vi "Create LVClass for Oneof.vi"(7 "Parent Message Typedef":refnum<vi>, 8 "error in (no error)":errorcluster, 9 "Message Elements":T1[](array[typedef]), 10 "Message Name":string, 11 "Library":refnum<vi>) -> (0 "error out":errorcluster, 3 "Library":refnum<vi>)   [LabVIEW 2019]
uses:
  TypeDefs/Message Element Metadata (Scripting).ctl
  TypeDefs/Message Element Type.ctl
  gRPC Template Creation Utility.lvlib
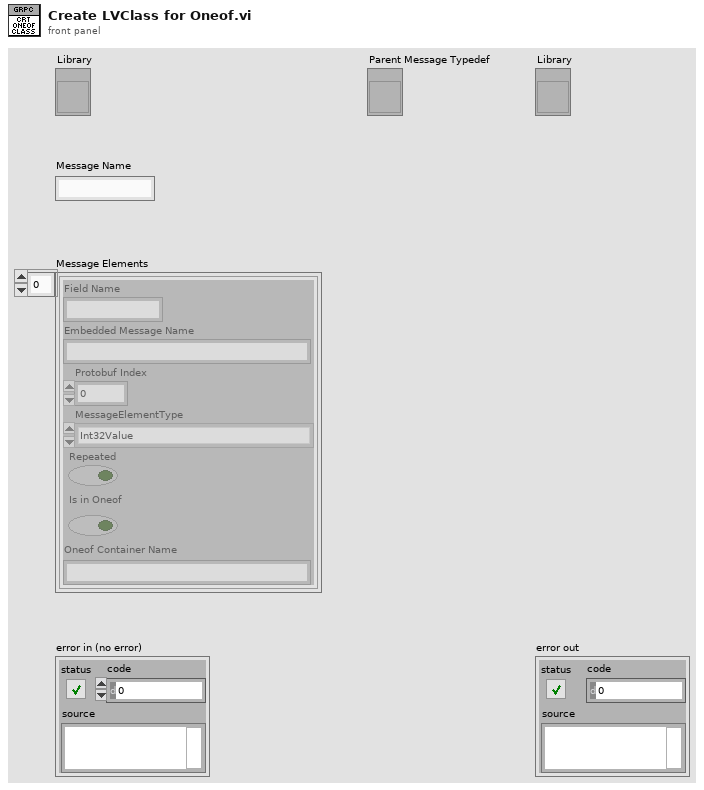
[diagram p1: front panel]
types:
  T1 = typedef "gRPC Template Creation Utility.lvlib/Message Element Metadata (Scripting).ctl" = cluster{"Field Name":string, "Embedded Message Name":string, "Protobuf Index":i32, "MessageElementType":T2, "Repeated":bool, "Is in Oneof":bool, "Oneof Container Name":string}
  T2 = typedef "gRPC Template Creation Utility.lvlib/Message Element Type.ctl" = enum32{"Int32Value", "FloatValue", "DoubleValue", "BoolValue", "StringValue", "MessageValue", "Int64Value", "UInt32Value", "UInt64Value", "EnumValue", "Bytes", "Fixed64", "Fixed32", "SFixed64", "SFixed32", "SInt64", "SInt32"}
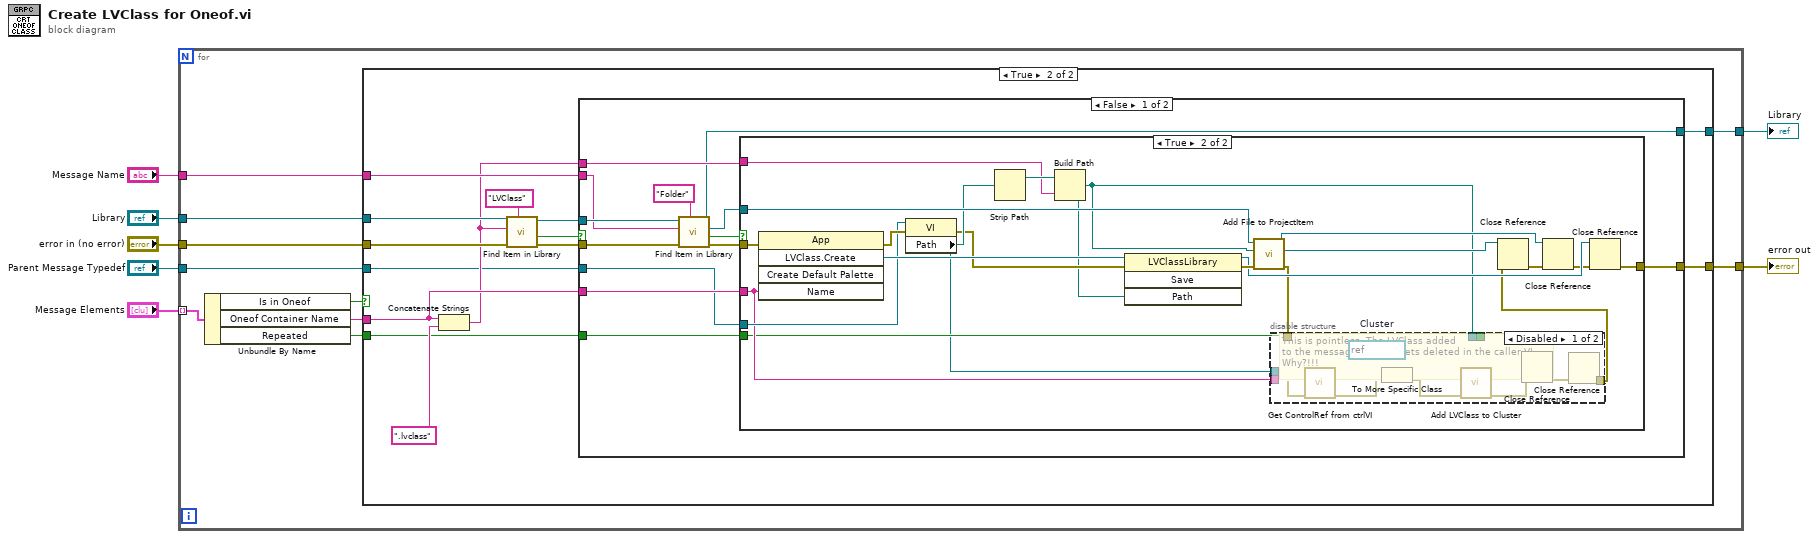
[diagram p0: block diagram]
diagram:
  n1 = for {
    tunnel: "Message Elements" -> [w17] mode=indexing
    tunnel: "error in (no error)" -> [w14]
    tunnel: [w13] -> w5
    tunnel: "Message Name" -> [w12]
    tunnel: "Library" -> [w11]
    tunnel: [w10] -> w2
    tunnel: "Parent Message Typedef" -> [w9]
    n2 = Unbundle By Name(w17) -> ("Is in Oneof"=w15:bool, "Oneof Container Name"=w16:string, "Repeated"=w8:bool)
    n3 = case shown="True" w15 {
      tunnel: [w19 w33] -> w13
      tunnel: w16 -> [_ w32]
      tunnel: w14 -> [w19 w29]
      tunnel: w12 -> [_ w31]
      tunnel: w11 -> [w18 w28]
      tunnel: [w18 w30] -> w10
      tunnel: w9 -> [_ w21]
      tunnel: w8 -> [_ w20]
      frame False {
      }
      frame True {
        n4 = Concatenate Strings(w32, ".lvclass" ("string")) -> (w25:string)
        n5 = call "Find Item in Library.vi"("Item Type"="LVClass", "error in (no error)"=w29, "Item Name"=w25, "Library item in"=w28) -> ("error out"=w23:errorcluster, "Found?"=w22:bool, "Library item out"=w27:refnum<vi>)  [unwired: 4 in, 1 out]
        n6 = case shown="False" w22 {
          tunnel: [w42 w86] -> w33
          tunnel: w32 -> [w41 _]
          tunnel: w31 -> [w36 _]
          tunnel: [w37 w87] -> w30
          tunnel: w27 -> [w38 w87]
          tunnel: w25 -> [w40 _]
          tunnel: w23 -> [w39 w86]
          tunnel: w21 -> [w35 _]
          tunnel: w20 -> [w34 _]
          frame False {
            n7 = call "Find Item in Library.vi"("Item Type"="Folder", "error in (no error)"=w39, "Item Name"=w36, "Library item in"=w38) -> ("error out"=w44:errorcluster, "Found?"=w43:bool, "Project Item (Library Item)"=w46:refnum<vi>, "Library item out"=w37:refnum<vi>)  [unwired: 4 in]
            n8 = case shown="True" w43 {
              tunnel: w41 -> [_ w52]
              tunnel: w46 -> [_ w66]
              tunnel: [w47 w54] -> w42
              tunnel: w44 -> [w47 w63]
              tunnel: w40 -> [_ w64]
              tunnel: w35 -> [_ w60]
              tunnel: w34 -> [_ w50]
              frame False {
                # "Container message should have been created already."
              }
              frame True {
                n9 = invoke class="App" method="LVClass.Create"(error in=w63, "Name"=w52) -> (error out=w62:errorcluster, "LVClass.Create"=w68:refnum<vi>)  [unwired: 3 in, 3 out]
                n10 = property class="VI"(reference=w60, error in=w62) -> (reference out=w49:refnum<vi>, error out=w59:errorcluster, "Path"=w61:path)
                n11 = Strip Path(path=w61) -> (stripped path=w67:path)  [unwired: 1 out]
                n12 = Build Path(base path=w67, name or relative path=w64) -> (appended path=w51:path)
                n13 = invoke class="LVClassLibrary" method="Save"(reference=w68, error in=w59, "Path"=w51) -> (reference out=w56:refnum<vi>, error out=w65:errorcluster)  [unwired: 1 in, 2 out]
                n14 = call "Add File to ProjectItem.vi"("error in (no error)"=w65, "File Path"=w51, "ProjectItem in"=w66) -> ("error out"=w48:errorcluster, "Added File ref"=w69:refnum<vi>, "ProjectItem out"=w57:refnum<vi>)  [unwired: 6 in]
                n15 = disable-structure shown="Disabled" {
                  disable-tunnel: [w82 w85] -> w53
                  disable-tunnel: w52 -> [w79 _]
                  disable-tunnel: w51 -> [w78 _]
                  disable-tunnel: w50 -> [w77 _]
                  disable-tunnel: w49 -> [w73 _]
                  disable-tunnel: w48 -> [w72 w85]
                  frame Disabled {
                    w84 = refnum<vi> refnum  # Cluster
                    # "This is pointless. The LVClass added\nto the message typedef gets deleted in the caller VI.\nWhy?!!!"
                    n16 = call "Get ControlRef from ctrlVI.vi"("error in (no error)"=w72, "VI ref in"=w73) -> ("error out"=w70:errorcluster, "Control ref out"=w71:refnum<vi>)  [unwired: 7 in, 1 out]
                    n17 = To More Specific Class(target class=w84, reference=w71, error in=w70) -> (specific class reference=w81:refnum<vi>, error out=w80:errorcluster)
                    n18 = call "Add LVClass to Cluster.vi"("isArray (F)"=w77, "LVClass path"=w78, "error in (no error)"=w80, "Field Name"=w79, "Owning cluster ref in"=w81) -> ("error out"=w74:errorcluster, "Control ref out"=w75:refnum<vi>, "Owning cluster ref out"=w76:refnum<vi>)  [unwired: 4 in]
                    n19 = Close Reference(reference=w76, error in (no error)=w74) -> (error out=w83:errorcluster)
                    n20 = Close Reference(reference=w75, error in (no error)=w83) -> (error out=w82:errorcluster)
                  }
                  frame Enabled {
                  }
                }
                n21 = Close Reference(reference=w69, error in (no error)=w53) -> (error out=w58:errorcluster)
                n22 = Close Reference(reference=w57, error in (no error)=w58) -> (error out=w55:errorcluster)
                n23 = Close Reference(reference=w56, error in (no error)=w55) -> (error out=w54:errorcluster)
              }
            }
          }
          frame True {
          }
        }
      }
    }
  }
  "error out" <- w5
  "Library" <- w2
